vi "BuildMethodCall.vi"(9 "params":string[](array[string]), 11 "methodName":string) -> (3 "XML":string)   [LabVIEW 2012]
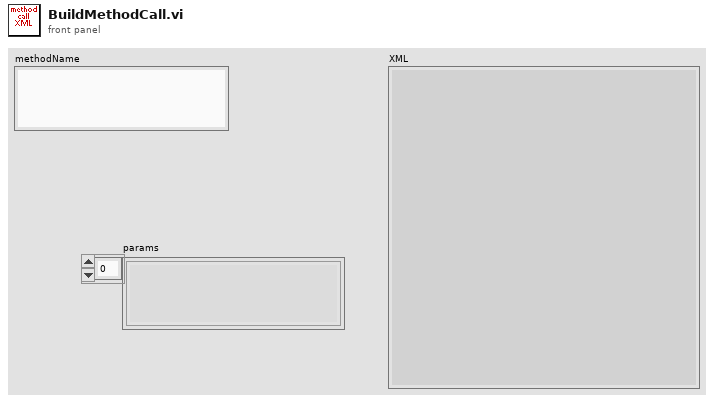
[diagram p1: front panel]
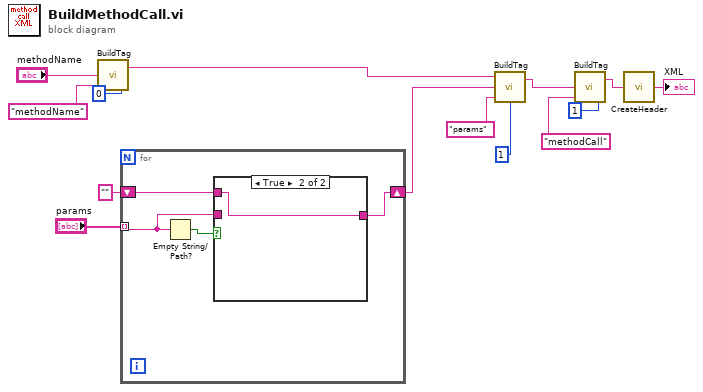
[diagram p0: block diagram]
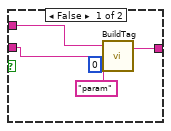
[diagram p2: hidden frame]
diagram:
  n1 = call <userlib>:"BuildTag.vi"("Indent"=i8 0, "tag"="methodName", "value"="methodName") -> ("string out"=w7:string)  [unwired: 1 in]
  n2 = for {
    tunnel: "params" -> [w15] mode=indexing
    shift-right: [w17] -> w2
    shift-left: "" ("string out") -> [w18]
    n3 = Empty String/Path?(string/path=w15) -> (empty?=w16:bool)
    n4 = case shown="True" w16 {
      tunnel: w18 -> [w23 w24]
      tunnel: [w22 w24] -> w17
      tunnel: w15 -> [w19 _]
      frame False {
        n5 = call <userlib>:"BuildTag.vi"("Indent"=i8 0, "tag"="param", "value"=w19, "string in"=w23) -> ("string out"=w22:string)
      }
      frame True {
      }
    }
  }
  n6 = call <userlib>:"BuildTag.vi"("Indent"=i8 1, "tag"="params", "value"=w2, "string in"=w7) -> ("string out"=w6:string)
  n7 = call <userlib>:"BuildTag.vi"("Indent"=i8 1, "tag"="methodCall", "value"=w6) -> ("string out"=w13:string)  [unwired: 1 in]
  n8 = call <userlib>:"CreateHeader.vi"("Content"=w13) -> ("XML"=→"XML":string)
